vi "Day 22-Part 2.vi"() -> ()   [LabVIEW 2021]
uses:
  <vilib>/Utility/file.llb/Read Delimited Spreadsheet (string).vi
panel:
  out "Map":map{i64[], i64}(c390)
  out "size":i32
  out "Cubes On":i64
  in  "Input File":enum32{"example input", "input"}(radio)
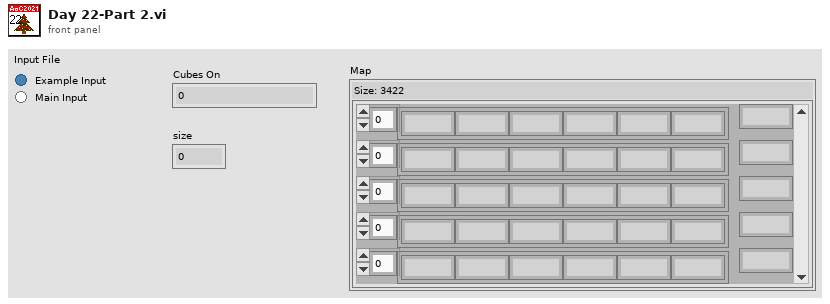
[diagram p1: front panel]
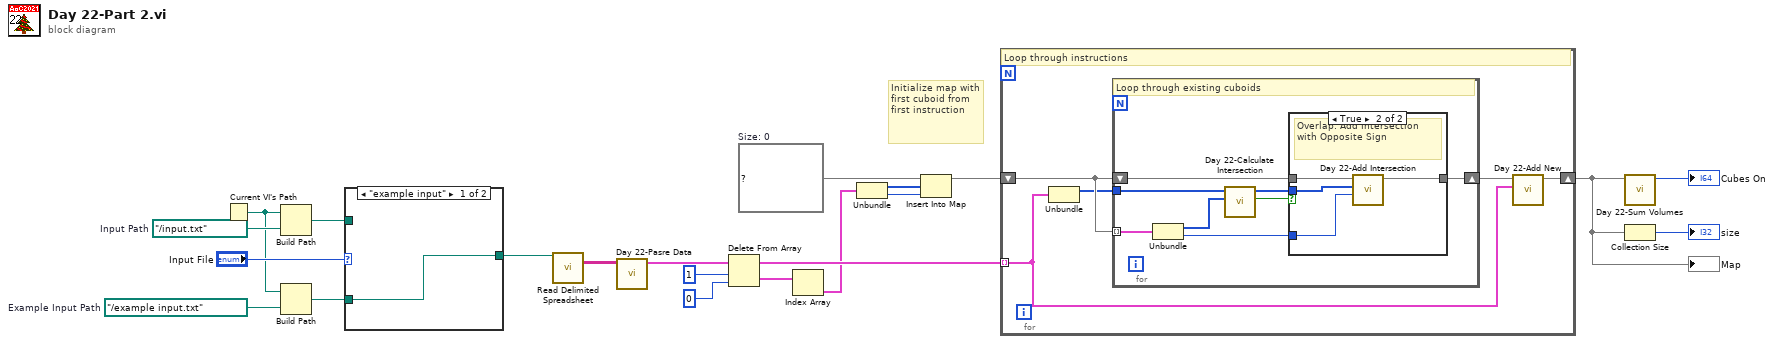
[diagram p0: block diagram]
diagram:
  w8 = map{i64[], i64} {}  # Size: 0
  w20 = path "../example input.txt"  # Example Input Path
  w21 = path "../input.txt"  # Input Path
  # "Initialize map with first cuboid from first instruction"
  n1 = Current VI's Path() -> (path=w15:path)
  n2 = Build Path(base path=w15, name or relative path=w21) -> (appended path=w18:path)
  n3 = Build Path(base path=w15, name or relative path=w20) -> (appended path=w17:path)
  n4 = case shown="\"example input\"" "Input File" {
    tunnel: w18 -> [_ w23]
    tunnel: w17 -> [w22 _]
    tunnel: [w22 w23] -> w16
    frame "example input" {
    }
    frame "input" {
    }
  }
  n5 = call-poly <vilib>:"Read Delimited Spreadsheet.vi"("file path (dialog if empty)"=w16) -> ("all rows"=w1:string[][])  [unwired: 9 in, 5 out]
  n6 = call "Day 22-Pasre Data.vi"("Data in"=w1) -> ("Instructions out"=w14:cluster{i64[], i64}[])  [unwired: 10 in]
  n7 = Delete From Array(array=w14, length=1, index=0) -> (deleted portion=w10:cluster{i64[], i64}[], array with subset deleted=w13:cluster{i64[], i64}[])
  n8 = Index Array(array=w10) -> (element=w6:cluster{i64[], i64})  [unwired: 1 in]
  n9 = Unbundle(w6) -> (w5:i64[], w4:i64)
  n10 = Insert Into Map(map in=w8, key=w5, value=w4) -> (map out=w7:map{i64[], i64})  [unwired: 2 out]
  n11 = for {
    tunnel: w13 -> [w24] mode=indexing
    shift-right: [w27] -> w3
    shift-left: w7 -> [w26]
    # "Loop through instructions"
    n12 = Unbundle(w24) -> (w25:i64[])  [unwired: 1 out]
    n13 = for {
      tunnel: w25 -> [w29]
      shift-right: [w36] -> w28
      shift-left: w26 -> [w35]
      tunnel: w26 -> [w34] mode=indexing
      # "Loop through existing cuboids"
      n14 = Unbundle(w34) -> (w30:i64[], w33:i64)
      n15 = call "Day 22-Calculate Intersection.vi"("Existing in"=w30, "New in"=w29) -> ("Is there Overlap?"=w31:bool, "Intersection out"=w32:i64[])  [unwired: 8 in]
      n16 = case shown="True" w31 {
        tunnel: w35 -> [w37 w41]
        tunnel: [w37 w40] -> w36
        tunnel: w33 -> [_ w38]
        tunnel: w32 -> [_ w39]
        frame False {
          # "No Overlap"
        }
        frame True {
          # "Overlap. Add Intersection with Opposite Sign"
          n17 = call "Day 22-Add Intersection.vi"("Sign"=w38, "Intersection in"=w39, "Map in"=w41) -> ("Map out"=w40:map{i64[], i64})  [unwired: 8 in]
        }
      }
    }
    n18 = call "Day 22-Add New.vi"("Instruction in"=w24, "Map in"=w28) -> ("Map out"=w27:map{i64[], i64})  [unwired: 9 in]
  }
  "Map" <- w3
  n19 = call "Day 22-Sum Volumes.vi"("Map"=w3) -> ("Volumn \"On\""=→"Cubes On":i64)  [unwired: 10 in]
  n20 = Collection Size(1:w3) -> (0:→"size":i32)
